vi "OnButton-TimedSequentialPress-Demo.vi"() -> ()   [LabVIEW 2015]
panel:
  in  "Trigger":bool
  out "Remaining":u8
  in  "Trigger Count":u8=2
  out "Triggered":bool
  in  "Timeout (ms)":u32=2500
  out "Timeout":u32
  out "Armed":bool
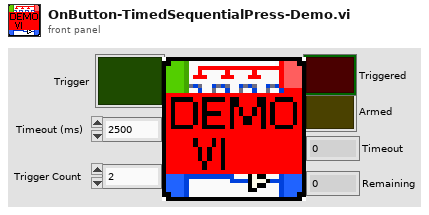
[diagram p1: front panel]
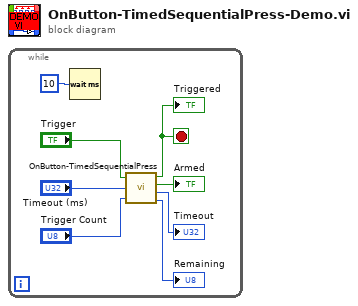
[diagram p0: block diagram]
diagram:
  n1 = while {
    stop <- w4 stop-if-true
    n2 = Wait (ms)(milliseconds to wait=u32 10) -> ()  [unwired: 1 out]
    n3 = call "OnButton-TimedSequentialPress.vi"("Trigger"="Trigger", "Timeout (ms)"="Timeout (ms)", "Trigger Count"="Trigger Count") -> ("Triggered"=w4:bool, "Armed"=→"Armed":bool, "Timeout"=→"Timeout":u32, "Remaining"=→"Remaining":u8)
    "Triggered" <- w4
  }
